vi "HackyNICard3.vi"() -> ()   [LabVIEW 2013]
uses:
  <vilib>/DAQmx/write.llb/DAQmx Write (Analog 2D DBL NChan NSamp).vi
  <vilib>/DAQmx/configure/timing.llb/DAQmx Timing (Sample Clock).vi
  <vilib>/DAQmx/miscellaneous.llb/DAQmx Fill In Error Info.vi
panel:
  out "error out":errorcluster
  in  "Clock line":tag
  out "Array Out":dbl[][](array[numeric])
  in  "Channel Values":cluster{"Channel":refnum<k21>, "Array":dbl[]}[](array[cluster])
  in  "stop":bool
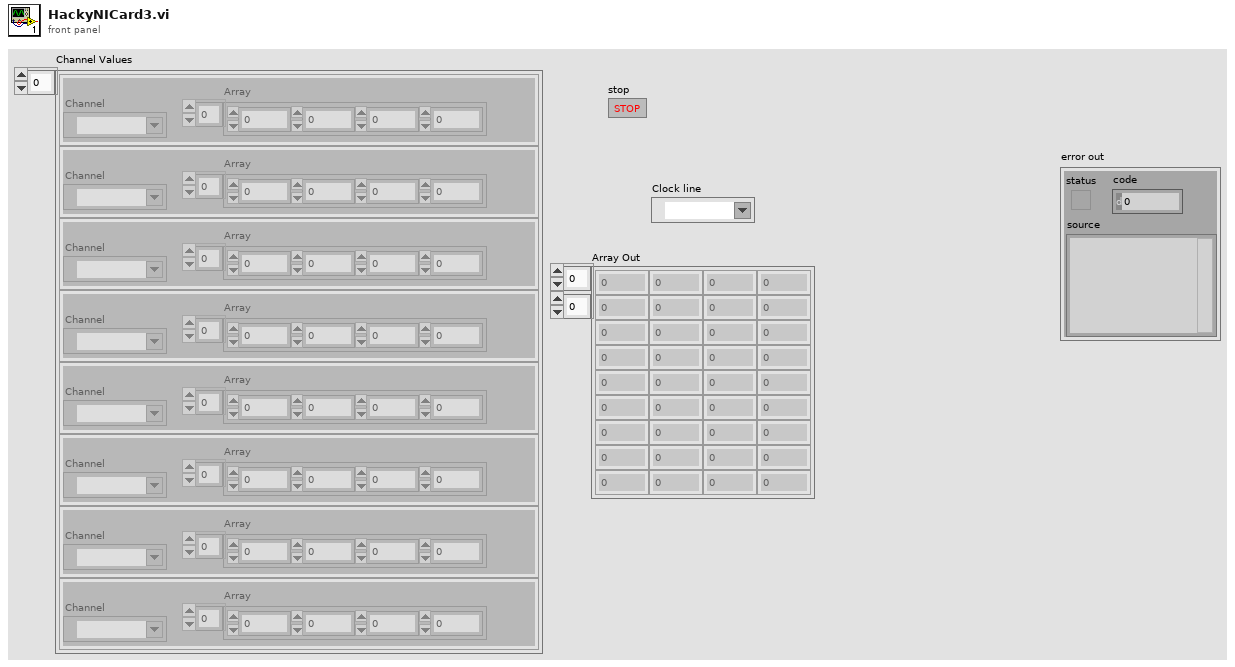
[diagram p1: front panel]
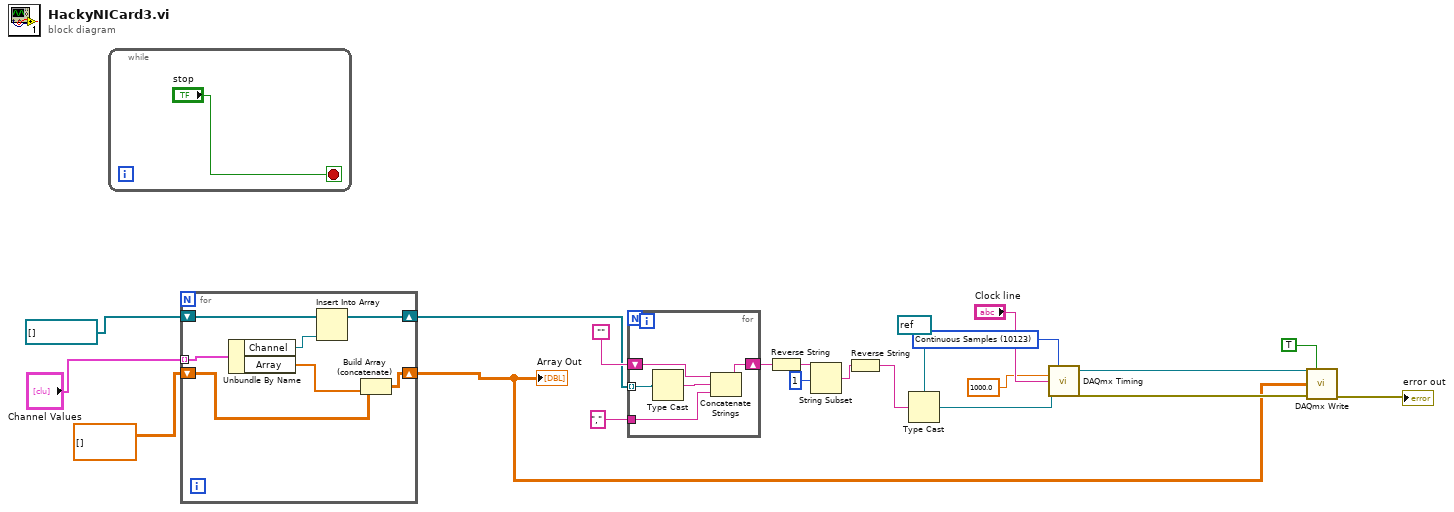
[diagram p0: block diagram]
diagram:
  w8 = 10123 items=["Finite Samples"=10178, "Continuous Samples"=10123, "Hardware Timed Single Point"=12522] ("sample mode")
  n1 = while {
    stop <- "stop" stop-if-true
  }
  n2 = for {
    tunnel: "Channel Values" -> [w29] mode=indexing
    shift-right: [w26] -> w1
    shift-left: refnum<k21>[] [] ("array") -> [w27]
    shift-right: [w25] -> w2
    shift-left: dbl[][] [] -> [w24]
    n3 = Unbundle By Name(w29) -> ("Channel"=w28:refnum<k21>, "Array"=w23:dbl[])
    n4 = Insert Into Array(array=w27, new element=w28) -> (w26:refnum<k21>[])  [unwired: 1 in]
    n5 = Build Array (concatenate)(w24, w23) -> (w25:dbl[][])
  }
  "Array Out" <- w2
  n6 = for {
    tunnel: w1 -> [w34] mode=indexing
    shift-right: [w31] -> w15
    shift-left: "" -> [w33]
    tunnel: "," -> [w32]
    n7 = Type Cast(x=w34) -> (*(type *) &x=w30:string)  [unwired: 1 in]
    n8 = Concatenate Strings(w33, w30, w32) -> (w31:string)
  }
  n9 = Reverse String(1:w15) -> (0:w14:string)
  n10 = String Subset(string=w14, offset (0)=1) -> (substring=w13:string)  [unwired: 1 in]
  n11 = Reverse String(1:w13) -> (0:w11:string)
  n12 = Type Cast(type=refnum<k21> refnum ("DAQmx Global Channel"), x=w11) -> (*(type *) &x=w9:refnum<k21>)
  n13 = call-poly <vilib>:"DAQmx Timing.vi"("task/channels in"=w9, "sample mode"=w8, "rate"=1000.0, "source"="Clock line") -> ("task out"=w7:refnum<k21>, "error out"=w6:errorcluster)  [unwired: 10 in]
  n14 = call-poly <vilib>:"DAQmx Write.vi"("task/channels in"=w7, "auto start"=TRUE, "data"=w2, "error in"=w6) -> ("error out"=→"error out":errorcluster)  [unwired: 9 in, 2 out]
